vi "Pre Launch Init.vi"(11 "Caller in":refnum<class "Actor.lvclass">) -> (0 "error out":errorcluster, 3 "Caller out":refnum<class "Actor.lvclass">)   [LabVIEW 2020, in "Actor.lvlib" / "Actor.lvclass"]
doc: "(<B>Filename</B>: Actor Framework.lvlib:Actor.lvclass:Pre Launch Init.vi)\n\nDefines behavior that occurs after the Launch Nested Actor method is invoked but before the actor's Actor Core method begins running.\n\nBy default, this method does nothing. A descendant class may override it to define behavior."
uses:
  Actor.lvclass
  C:/Program Files/National Instruments/LabVIEW 2020/vi.lib/ActorFramework/Actor/Actor.lvclass
  Actor.lvclass/Actor.ctl
  <vilib>/ActorFramework/Actor/Actor.lvclass/Actor.ctl
  <vilib>/ActorFramework/Message Enqueuer/Message Enqueuer.lvclass/Message Enqueuer.ctl
  <vilib>/ActorFramework/Message Enqueuer/Init from Existing Queue.vi
  <vilib>/ActorFramework/Actor/Actor.lvclass
  <vilib>/ActorFramework/Message Enqueuer/Message Enqueuer.lvclass
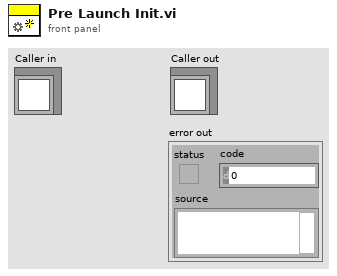
[diagram p1: front panel]
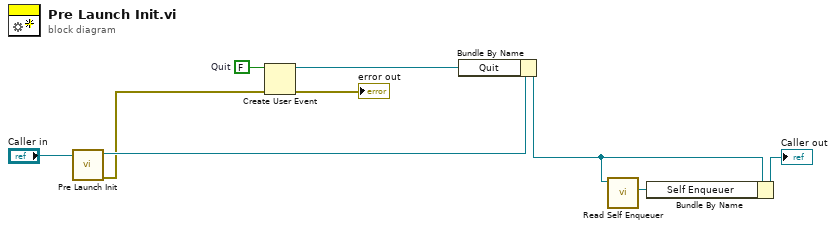
[diagram p0: block diagram]
diagram:
  w9 = FALSE  # Quit
  n1 = call-parent "Pre Launch Init.vi"("Actor in"="Caller in") -> ("error out"=w2:errorcluster, "Actor out"=w4:refnum<class "Actor.lvclass">)  [unwired: 9 in]
  n2 = Create User Event(user event datatype=w9, error in=w2) -> (user event=w8:refnum<user-event>, error out=→"error out":errorcluster)
  n3 = Bundle By Name(cluster=w4, "Quit"=w8) -> (w3:refnum<class "Actor.lvclass">)
  n4 = call <vilib>:"Read Self Enqueuer.vi"("Actor"=w3) -> ("Self Enqueuer"=w6:refnum<class "Message Enqueuer.lvclass">)  [unwired: 10 in]
  n5 = Bundle By Name(cluster=w3, "Self Enqueuer"=w6) -> (→"Caller out":refnum<class "Actor.lvclass">)
